vi "Config_Image_Read_MapPath.vi"(8 "error in (no error)":errorcluster) -> (0 "error out":errorcluster)   [LabVIEW 2020]
uses:
  <vilib>/Utility/config.llb/Read Key (Path).vi
  <vilib>/Utility/config.llb/NI_LVConfig.lvlib
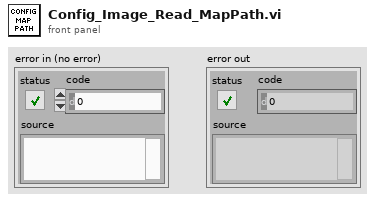
[diagram p1: front panel]
types:
  T1 = typedef "Image_Cluster.ctl" = cluster{"Detector_info":cluster{"No. of detectors":dbl, "Detector_Array":string[][], "Detector_Array_Numeric":dbl[][]}, "Corner_info":cluster{"Corner_Array":dbl[][]}, "ROI":cluster{"Corners":cluster{"Global Rectangle":i32[], "Contours":cluster{"ID":enum32{"External", "Internal"}, "Type":u32, "Coordinates":i32[]}[]}[], "Detectors":cluster{"Global Rectangle":i32[], "Contours":cluster{"ID":enum32{"External", "Internal"}, "Type":u32, "Coordinates":i32[]}[]}[]}, "Shape_Detect":cluster{"Match_score":dbl, "Curve Parameters":T2, "Match Options":T3, "Circle Descriptor":cluster{"Min Radius":dbl, "Max Radius":dbl}}, "Path":cluster{"Config":path, "Map":path}, "Map":cluster{"X_resolution":i32, "Y_resolution":i32, "Image":T5, "Image_colored":T5}, "Conversion_factor":dbl}
  T2 = typedef "IMAQ Curve Parameters.ctl" = cluster{"Extraction Mode":u32, "Edge Threshold":i32, "Edge Filter Size":u32, "Min Length":i32, "Row Search Step Size":i32, "Col Search Step Size":i32, "Max Endpoint Gap":i32, "Closed":bool, "Subpixel":bool}
  T3 = typedef "ShapeDetectionMatchOptions.ctl" = cluster{"Rotation":bool, "Scale":bool, "Occlusion":bool, "Range Settings":T4[]}
  T4 = typedef "IMAQ Match Range Setting.ctl" = cluster{"Match Constraints":u32, "Min":dbl, "Max":dbl}
  T5 = typedef "IMAQ Image.ctl" = refnum<image>
  T6 = typedef "NI_LVConfig.lvlib/Config Data RefNum.ctl" = refnum<k1>
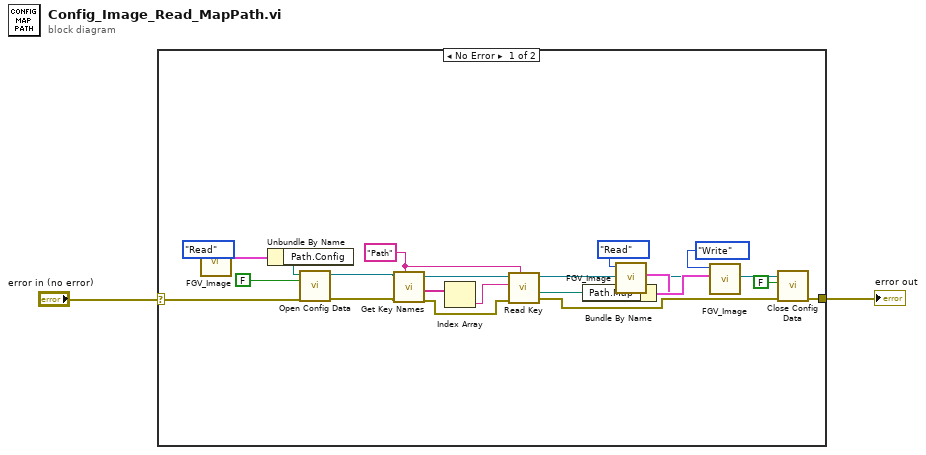
[diagram p0: block diagram]
diagram:
  n1 = case shown="No Error" "error in (no error)" {
    selector: "error in (no error)" -> [w13 w24]
    tunnel: [w23 w24] -> w2
    frame No Error {
      w7 = "Path"
      n2 = call "FGV_Image.vi"("Action"=enum16{"Read", "Write", ""}."Read") -> ("Image_Cluster_out"=w21:T1)  [unwired: 10 in]
      n3 = Unbundle By Name(w21) -> ("Path.Config"=w22:path)
      n4 = call <vilib>:"Open Config Data.vi"("error in (no error)"=w13, "create file if necessary (T)"=FALSE, "configuration file path"=w22) -> ("error out"=w12:errorcluster, "refnum"=w11:T6)  [unwired: 6 in, 1 out]
      n5 = call <vilib>:"Get Key Names.vi"("section"=w7, "error in (no error)"=w12, "refnum"=w11) -> ("error out"=w6:errorcluster, "key names"=w9:string[], "refnum out"=w10:T6)  [unwired: 5 in, 1 out]
      n6 = Index Array(array=w9) -> (element=w8:string)  [unwired: 1 in]
      n7 = call-poly <vilib>:"Read Key.vi"("section"=w7, "error in (no error)"=w6, "key"=w8, "refnum"=w10) -> ("error out"=w3:errorcluster, "value"=w4:path, "refnum out"=w5:T6)  [unwired: 4 in, 1 out]
      n8 = call "FGV_Image.vi"("Action"=enum16{"Read", "Write", ""}."Read") -> ("Image_Cluster_out"=w17:T1)  [unwired: 10 in]
      n9 = Bundle By Name(cluster=w17, "Path.Map"=w4) -> (w18:T1)
      n10 = call "FGV_Image.vi"("Image_Cluster_in"=w18, "Action"=enum16{"Read", "Write", ""}."Write") -> ()  [unwired: 9 in, 1 out]
      n11 = call <vilib>:"Close Config Data.vi"("error in (no error)"=w3, "write file if changed (T)"=FALSE ("write configuration file? (T)"), "refnum"=w5) -> ("error out"=w23:errorcluster)  [unwired: 8 out]
    }
    frame Error {
    }
  }
  "error out" <- w2
